vi "logic_gates.vi"() -> ()   [LabVIEW 2018]
panel:
  in  "Y":bool
  in  "X":bool
  out "EXNOR Output":bool
  out "XOR Output":bool
  out "OR Output":bool
  out "AND Output":bool
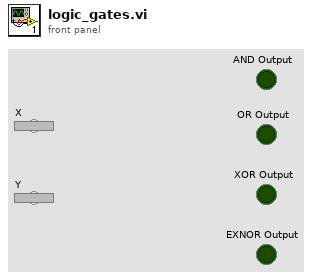
[diagram p1: front panel]
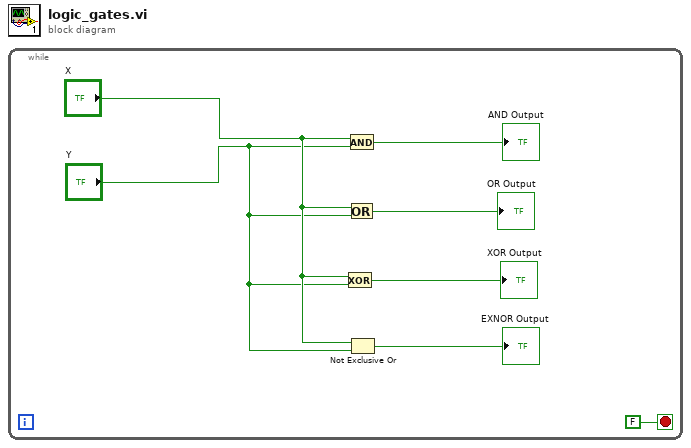
[diagram p0: block diagram]
diagram:
  n1 = while {
    stop <- FALSE stop-if-true
    n2 = Exclusive Or(1:"Y", 2:"X") -> (0:→"XOR Output":bool)
    n3 = And(x="X", y="Y") -> (x .and. y?=→"AND Output":bool)
    n4 = Or(x="X", y="Y") -> (x .or. y?=→"OR Output":bool)
    n5 = Not Exclusive Or(1:"Y", 2:"X") -> (0:→"EXNOR Output":bool)
  }
